vi "Find peak and build graph.vi"(9 "hour":i32, 10 "date":i32, 11 "data":dbl[][](array[numeric])) -> (0 "Average usage /hour":dbl format="%0.2f", 2 "XY Graph":cluster{"Y":dbl[], "Y":dbl[]}[](graph), 3 "Profile per day":dbl[][](graph), 4 "min index(es)":i32, 5 "max index(es)":i32, 6 "min value":dbl, 7 "max value":dbl)   [LabVIEW 2018]
uses:
  <vilib>/Analysis/NI_AALBase.lvlib
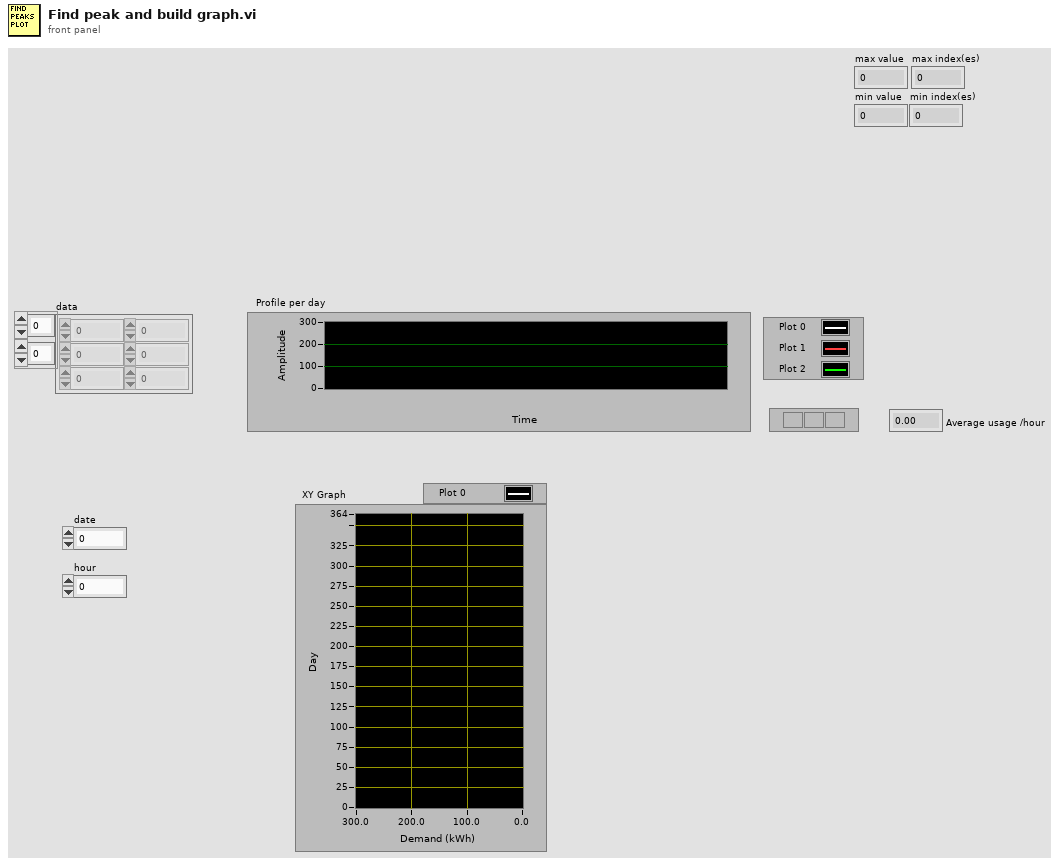
[diagram p1: front panel]
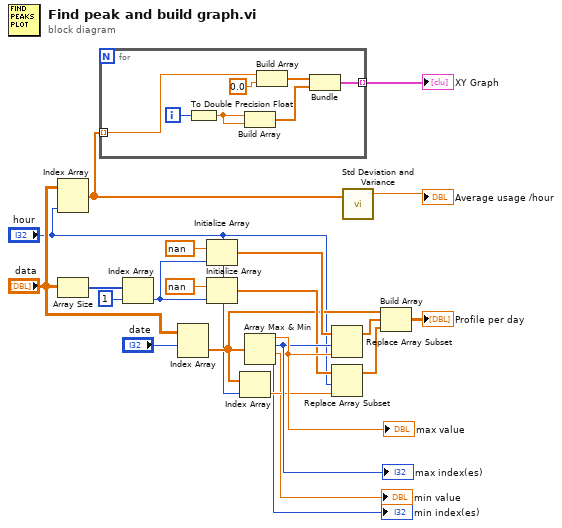
[diagram p0: block diagram]
diagram:
  n1 = Index Array(array="data", index (col)="hour") -> (element=w4:dbl[])  [unwired: 1 in]
  n2 = Array Size(array="data") -> (size(s)=w21:i32[])
  n3 = for {
    tunnel: w4 -> [w29] mode=indexing
    tunnel: [w24] -> w13 mode=indexing
    i -> [w23]
    n4 = To Double Precision Float(number=w23) -> (double precision float=w27:dbl)
    n5 = Build Array(w27, w27) -> (w25:dbl[])
    n6 = Build Array(w29, 0.0) -> (w26:dbl[])
    n7 = Bundle(w26, w25) -> (w24:cluster{dbl[], dbl[]})  [unwired: 1 in]
  }
  "XY Graph" <- w13
  n8 = Index Array(array=w21, index=1) -> (element=w11:i32)
  n9 = Index Array(array="data", index (row)="date") -> (element=w8:dbl[])  [unwired: 1 in]
  n10 = Initialize Array(nan, w11) -> (w9:dbl[])
  n11 = Initialize Array(nan, w11) -> (w10:dbl[])
  n12 = Index Array(array=w8, index="hour") -> (element=w6:dbl)
  n13 = Array Max & Min(array=w8) -> (max value=w19:dbl, max index (indices)=w16:i32, min value=→"min value":dbl, min index (indices)=→"min index(es)":i32)
  "max value" <- w19
  "max index(es)" <- w16
  n14 = Replace Array Subset(array=w9, new element=w19, index=w16) -> (w18:dbl[])
  n15 = Replace Array Subset(array=w10, new element=w6, index="hour") -> (w5:dbl[])
  n16 = call <vilib>:"Std Deviation and Variance.vi"("X"=w4) -> ("mean"=→"Average usage /hour":dbl)  [unwired: 1 in, 2 out]
  n17 = Build Array(w8, w18, w5) -> (→"Profile per day":dbl[][])
